vi "get engine name.vi"(8 "error in (no error)":errorcluster, 11 "engine in":refnum<class "Engine Parent Editor Node.lvclass">) -> (0 "error out":errorcluster, 2 "engine name":string, 3 "engine out":refnum<class "Engine Parent Editor Node.lvclass">)   [LabVIEW 2013, in "Shared Memory editor node.lvclass"]
uses:
  Shared Memory editor node.lvclass
  <vilib>/NI/DCAF/Tag Editor Core/Configuration Editor/Classes/Engine Parent/Engine Parent Editor Node.lvclass
  <vilib>/NI/DCAF/Tag Editor Core/Configuration Editor/Classes/Engine Parent/read engine configuration.vi
  <vilib>/NI/Configuration Framework/serializable configuration/get alias.vi
  <vilib>/NI/Module Execution Interface/Engine Configuration/engine configuration.lvclass
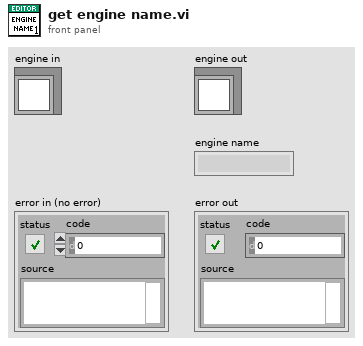
[diagram p1: front panel]
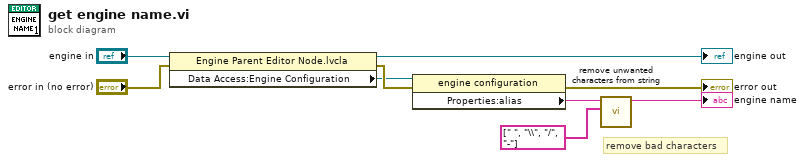
[diagram p0: block diagram]
diagram:
  # "remove bad characters"
  n1 = property class="Engine Parent Editor Node.lvcla"(reference="engine in", error in="error in (no error)") -> (reference out=→"engine out":refnum<class "Engine Parent Editor Node.lvclass">, error out=w9:errorcluster, "Data Access:Engine Configuration"=w4:refnum<class "engine configuration.lvclass">)
  n2 = property class="engine configuration"(reference=w4, error in=w9) -> (error out=→"error out":errorcluster, "Properties:alias"=w2:string)  [unwired: 1 out]
  n3 = call "remove unwanted characters from string.vi"("unwanted patterns/characters"=string[] [" ", "\\", "/", "-"], "string in"=w2) -> ("string out"=→"engine name":string)  [unwired: 9 in]
